vi "DHE_ReplaceMacroArgs_orig.vi"(9 "args":string[](array[string]), 10 "command in":string) -> (2 "comand out":string)   [LabVIEW 2016]
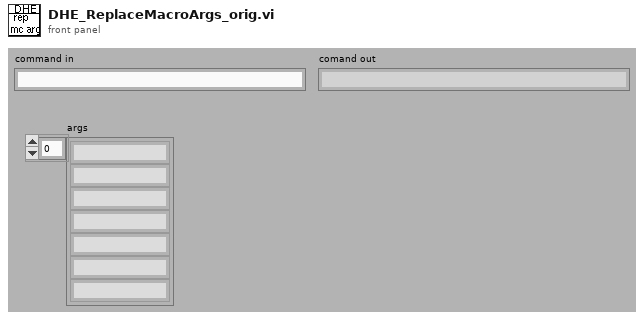
[diagram p1: front panel]
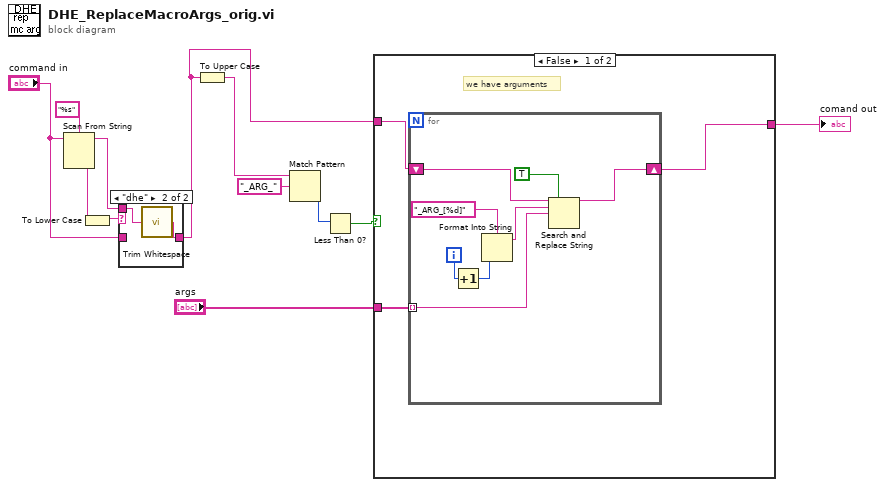
[diagram p0: block diagram]
diagram:
  n1 = Scan From String(format string="%s", input string="command in") -> (remaining string=w1:string, output 1=w5:string)  [unwired: 2 in, 3 out]
  n2 = To Lower Case(string=w5) -> (all lower case string=w4:string)
  n3 = case shown="\"dhe\"" w4 {
    tunnel: "command in" -> [w13 _]
    tunnel: [w13 w14] -> w2
    tunnel: w1 -> [_ w15]
    frame Default {
    }
    frame "dhe" {
      n4 = call <vilib>:"Trim Whitespace.vi"("string"=w15) -> ("trimmed string"=w14:string)  [unwired: 1 in]
    }
  }
  n5 = To Upper Case(1:w2) -> (0:w8:string)
  n6 = Match Pattern(string=w8, regular expression="_ARG_") -> (offset past match=w9:i32)  [unwired: 4 out]
  n7 = Less Than 0?(x=w9) -> (x < 0?=w7:bool)
  n8 = case shown="False" w7 {
    tunnel: w2 -> [w17 w27]
    tunnel: [w16 w27] -> w12
    tunnel: "args" -> [w18 _]
    frame False {
      # "we have arguments"
      n9 = for {
        tunnel: w18 -> [w24] mode=indexing
        shift-right: [w19] -> w16
        shift-left: w17 -> [w26]
        i -> [w23]
        n10 = Increment(x=w23) -> (x+1=w22:i32)
        n11 = Format Into String(format string="_ARG_[%d]", w22) -> (resulting string=w20:string)  [unwired: 2 in, 1 out]
        n12 = Search and Replace String(replace all?=TRUE ("replace all? (F)"), input string=w26, search string=w20, replace string=w24) -> (result string=w19:string)  [unwired: 1 in, 6 out]
      }
    }
    frame True {
      # "no arguments needed"
    }
  }
  "comand out" <- w12
